vi "Run Tx Measurement.vi"(0 "Refnum in":T2, 1 "Measurement":T1, 7 "Payload Length Mode":i32(ring)=1 items=["Manual", "Auto"], 9 "Payload Length (bytes)":i32, 11 "error in (no error)":errorcluster, 12 "Averaging Enabled":i32, 13 "Averaging Count":i32) -> (4 "Refnum out":T2, 15 "error out":errorcluster)   [LabVIEW 2025, in "Nordic nRF52 DK DTM Test.lvlib"]
uses:
  Nordic nRF52 DK DTM Test.lvlib
  <resource>/objmgr/RFmxBT.rc
  <vilib>/RFmx/RFInstr/mx/Support/RFmxInstrSupport.llb/niRFmx Instrument Handle.ctl
  Measurement.ctl
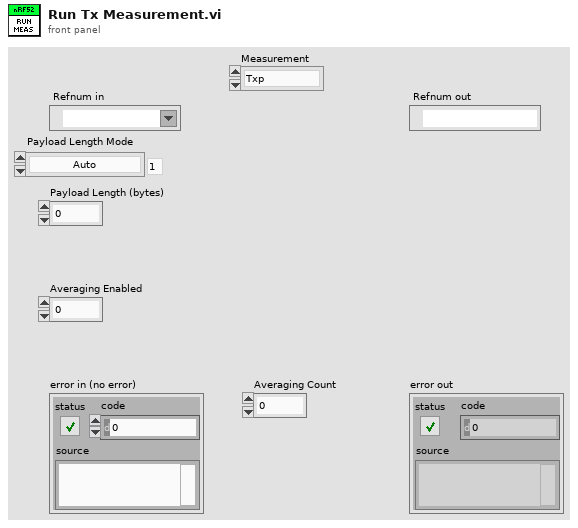
[diagram p1: front panel]
types:
  T1 = typedef "Nordic nRF52 DK DTM Test.lvlib/Measurement.ctl" = enum16{"Txp", "ACLR", "df1", "df2"}
  T2 = typedef "niRFmx Instrument Handle.ctl" = refnum<k21>
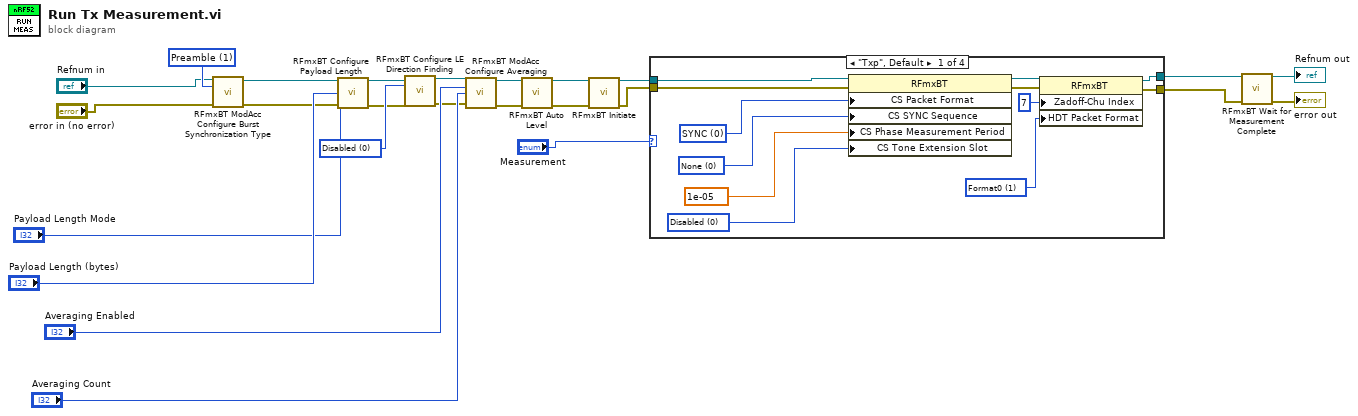
[diagram p0: block diagram]
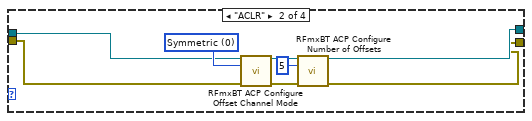
[diagram p2: hidden frame]
diagram:
  w11 = 1 items=["None", "Preamble", "Sync Word"] ("Burst Sync Type")
  w16 = 0 items=["Disabled", "Angle of Arrival", "Angle of Departure"] ("Direction Finding Mode")
  n1 = call <vilib>:"RFmxBT ModAcc Configure Burst Synchronization Type.vi"("Instrument Handle In"="Refnum in", "Burst Synchronization Type"=w11, "error in (no error)"="error in (no error)") -> ("Instrument Handle Out"=w9:refnum<k21>, "error out"=w10:errorcluster)  [unwired: 11 in]
  n2 = call <vilib>:"RFmxBT Configure Payload Length.vi"("Instrument Handle In"=w9, "Payload Length Mode"="Payload Length Mode", "Payload Length (bytes)"="Payload Length (bytes)", "error in (no error)"=w10) -> ("Instrument Handle Out"=w17:refnum<k21>, "error out"=w15:errorcluster)  [unwired: 10 in]
  n3 = call <vilib>:"RFmxBT Configure LE Direction Finding.vi"("Instrument Handle In"=w17, "Direction Finding Mode"=w16, "error in (no error)"=w15) -> ("Instrument Handle Out"=w18:refnum<k21>, "error out"=w19:errorcluster)  [unwired: 11 in]
  n4 = call <vilib>:"RFmxBT ModAcc Configure Averaging.vi"("Instrument Handle In"=w18, "Averaging Enabled"="Averaging Enabled", "Averaging Count"="Averaging Count", "error in (no error)"=w19) -> ("Instrument Handle Out"=w23:refnum<k21>, "error out"=w22:errorcluster)  [unwired: 10 in]
  n5 = call <vilib>:"RFmxBT Auto Level.vi"("Instrument Handle In"=w23, "error in (no error)"=w22) -> ("Instrument Handle Out"=w25:refnum<k21>, "error out"=w24:errorcluster)  [unwired: 11 in, 1 out]
  n6 = call <vilib>:"RFmxBT Initiate.vi"("Instrument Handle In"=w25, "error in (no error)"=w24) -> ("Instrument Handle Out"=w5:refnum<k21>, "error out"=w4:errorcluster)  [unwired: 11 in, 1 out]
  n7 = case shown="\"Txp\", Default" "Measurement" {
    tunnel: w5 -> [w37 w41 w47 w49]
    tunnel: w4 -> [w36 w40 w46 w48]
    tunnel: [w27 w39 w47 w49] -> w3
    tunnel: [w26 w38 w46 w48] -> w2
    frame "Txp", Default {
      w28 = 1 items=["Short Format", "Format0", "Format1"] ("HDT Packet Format")
      w32 = 0 items=["Disabled", "Enabled"] ("CS Tone Extension Slot")
      w33 = 1e-05 items=["10 us"=1e-05, "20 us"=2e-05, "40 us"=4e-05] ("CS Phase Measurement Period")
      w34 = 0 items=["None", "Sounding Sequence 32-bit", "Sounding Sequence 96-bit", "Payload Pattern"] ("CS SYNC Sequence")
      w35 = 0 items=["SYNC", "CS Tone", "CS Tone after SYNC", "CS Tone before SYNC"] ("CS Packet Format")
      n8 = property class="RFmxBT"(reference=w37, error in=w36, "CS Packet Format"=w35, "CS SYNC Sequence"=w34, "CS Phase Measurement Period"=w33, "CS Tone Extension Slot"=w32) -> (reference out=w31:refnum<k21>, error out=w30:errorcluster)
      n9 = property class="RFmxBT"(reference=w31, error in=w30, "Zadoff-Chu Index"=7, "HDT Packet Format"=w28) -> (reference out=w27:refnum<k21>, error out=w26:errorcluster)
    }
    frame "ACLR" {
      w45 = 0 items=["Symmetric", "In-band"] ("Offset Channel Mode")
      n10 = call <vilib>:"RFmxBT ACP Configure Offset Channel Mode.vi"("Instrument Handle In"=w41, "Offset Channel Mode"=w45, "error in (no error)"=w40) -> ("Instrument Handle Out"=w43:refnum<k21>, "error out"=w44:errorcluster)  [unwired: 11 in]
      n11 = call <vilib>:"RFmxBT ACP Configure Number of Offsets.vi"("Instrument Handle In"=w43, "Number of Offsets"=5, "error in (no error)"=w44) -> ("Instrument Handle Out"=w39:refnum<k21>, "error out"=w38:errorcluster)  [unwired: 11 in]
    }
    frame "df1" {
    }
    frame "df2" {
    }
  }
  n12 = call <vilib>:"RFmxBT Wait for Measurement Complete.vi"("Instrument Handle In"=w3, "error in (no error)"=w2) -> ("Instrument Handle Out"=→"Refnum out":refnum<k21>, "error out"=→"error out":errorcluster)  [unwired: 12 in]
